vi "OffsetRect by H and Rect Array.vi"(8 "错误输入":errorcluster, 10 "h":i16, 11 "Rect Array":T1(array[cluster])) -> (0 "错误输出":errorcluster, 3 "OffsetRect Array":T1(array[cluster]))   [LabVIEW 2012, in "Rect Tools.lvlib"]
uses:
  Rect Tools.lvlib
  OffsetRect by HV and Rect.vi
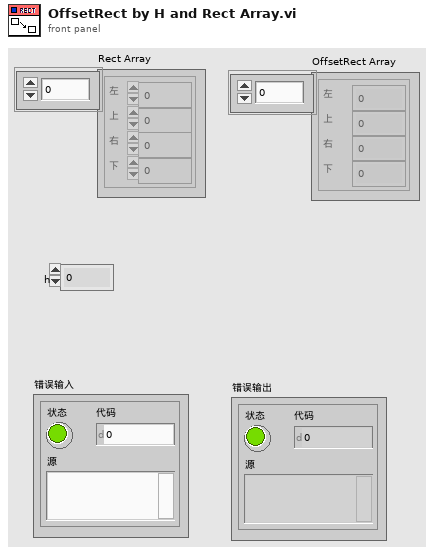
[diagram p1: front panel]
types:
  T1 = cluster{"left":i16, "top":i16, "right":i16, "bottom":i16}[]
  T2 = cluster{"left":i16, "top":i16, "right":i16, "bottom":i16}
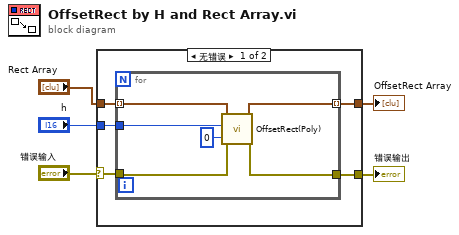
[diagram p0: block diagram]
diagram:
  n1 = case shown="无错误" "错误输入" {
    selector: "错误输入" -> [w7 w18]
    tunnel: [w6 w18] -> w4
    tunnel: "h" -> [w9 _]
    tunnel: "Rect Array" -> [w10 w17]
    tunnel: [w8 w17] -> w1
    frame No Error {
      n2 = for {
        tunnel: w10 -> [w15] mode=indexing
        tunnel: w9 -> [w16]
        tunnel: [w14] -> w8 mode=indexing
        tunnel: w7 -> [w13]
        tunnel: [w12] -> w6
        n3 = call-poly "OffsetRect(Poly).vi"("错误输入"=w13, "v"=i16 0, "h"=w16, "rect"=w15) -> ("错误输出"=w12:errorcluster, "offset rect"=w14:T2)  [unwired: 6 in]
      }
    }
    frame Error {
    }
  }
  "错误输出" <- w4
  "OffsetRect Array" <- w1
